vi "SerialArduino.vi"() -> ()   [LabVIEW 2019]
uses:
  96367c49-4912-4b9a-9665-363ed8841c2b.vi
  <vilib>/Instr/_visa.llb/VISA Configure Serial Port (Instr).vi
panel:
  out "return count":u32
  out "read buffer 2":string
  in  "Combo Box":string(combo)
  in  "stop":bool
  in  "Do Command":bool
  out "Result":dbl
  in  "Inputs":dbl[](array[numeric])
  out "error out":errorcluster
  out "read buffer":string
  in  "VISA resource name":refnum<visa-resource-name>
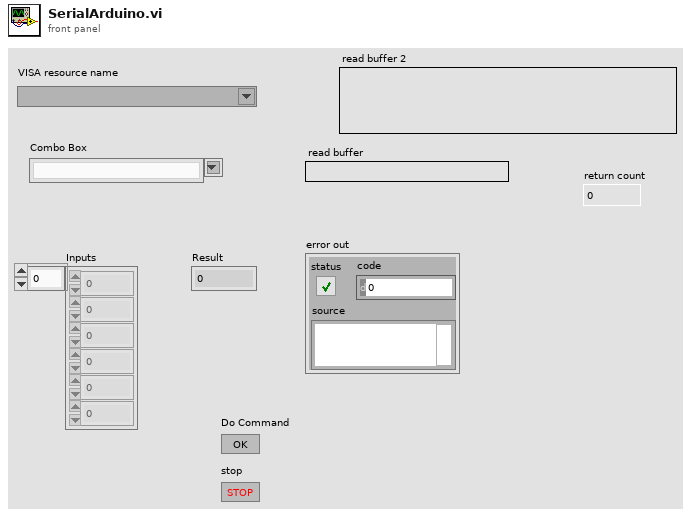
[diagram p1: front panel]
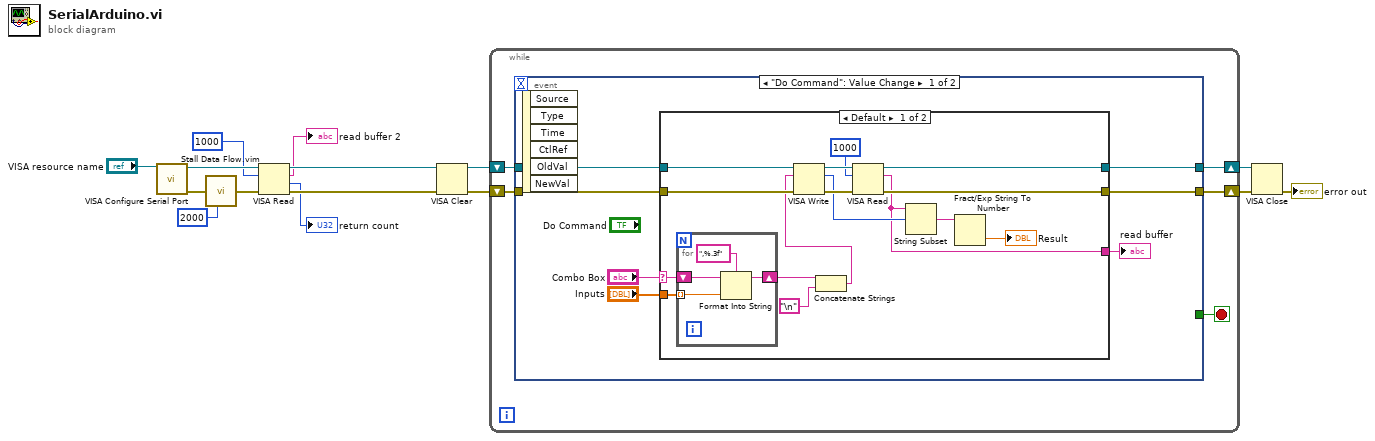
[diagram p0: block diagram]
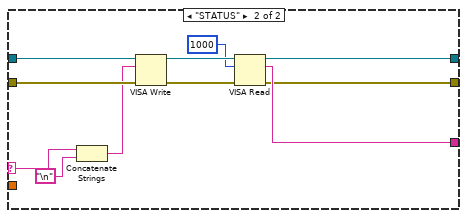
[diagram p2: hidden frame]
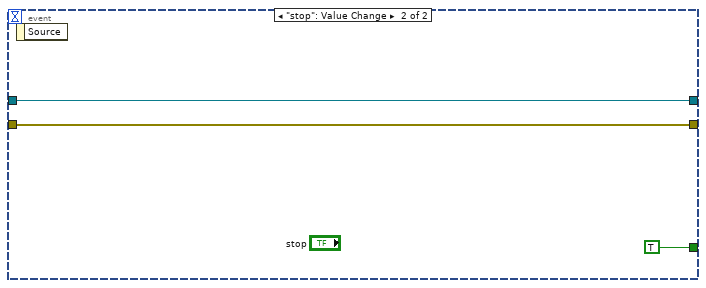
[diagram p3: hidden frame]
diagram:
  n1 = call-poly "VISA Configure Serial Port"("VISA resource name"="VISA resource name") -> ("VISA resource name out"=w5:refnum<visa-resource-name>, "error out"=w15:errorcluster)  [unwired: 13 in]
  n2 = call "Stall Data Flow.vim"("value in"=w15, "milliseconds to wait"=u32 2000) -> ("value out"=w8:errorcluster)  [unwired: 1 out]
  n3 = VISA Read(VISA resource name=w5, byte count=u32 1000, error in (no error)=w8) -> (VISA resource name out=w4:refnum<visa-resource-name>, read buffer=→"read buffer 2":string, return count=→"return count":u32, error out=w6:errorcluster)
  n4 = VISA Clear(VISA resource name=w4, error in (no error)=w6) -> (VISA resource name out=w14:refnum<visa-resource-name>, error out=w13:errorcluster)
  n5 = while {
    shift-right: [w18] -> w12
    shift-left: w14 -> [w20]
    shift-right: [w17] -> w11
    shift-left: w13 -> [w19]
    stop <- w16 stop-if-true
    n6 = event shown="[0] \"Do Command\": Value Change" {
      selector: _ -> [_ _]
      dyn-events: _ -> [_ _]
      timeout: _ -> [_ _]
      tunnel: w20 -> [w27 w60]
      tunnel: w19 -> [w26 w59]
      tunnel: [w25 w60] -> w18
      tunnel: [w24 w59] -> w17
      tunnel: [_ TRUE] -> w16
      event "Do Command": Value Change {
        n7 = event-data() -> ()  [unwired: 1 in, 6 out]
        n8 = case shown="Default" "Combo Box" {
          selector: "Combo Box" -> [w30 w50]
          tunnel: w27 -> [w43 w55]
          tunnel: w26 -> [w42 w54]
          tunnel: [w38 w51] -> w25
          tunnel: [w37 w52] -> w24
          tunnel: [w29 w53] -> w22
          tunnel: "Inputs" -> [w28 _]
          frame Default {
            n9 = for {
              shift-right: [w45] -> w36
              shift-left: w30 -> [w46]
              tunnel: w28 -> [w44] mode=indexing
              n10 = Format Into String(format string=",%.3f", initial string=w46, w44) -> (resulting string=w45:string)  [unwired: 1 in, 1 out]
            }
            n11 = Concatenate Strings(w36, "\n") -> (w34:string)
            n12 = VISA Write(VISA resource name=w43, write buffer=w34, error in (no error)=w42) -> (VISA resource name out=w41:refnum<visa-resource-name>, return count=w33:u32, error out=w40:errorcluster)
            n13 = VISA Read(VISA resource name=w41, byte count=u32 1000, error in (no error)=w40) -> (VISA resource name out=w38:refnum<visa-resource-name>, read buffer=w29:string, error out=w37:errorcluster)  [unwired: 1 out]
            n14 = String Subset(string=w29, offset (0)=w33) -> (substring=w32:string)  [unwired: 1 in]
            n15 = Fract/Exp String To Number(string=w32) -> (number=→"Result":dbl)  [unwired: 3 in, 1 out]
          }
          frame "STATUS" {
            n16 = Concatenate Strings(w50, "\n") -> (w49:string)
            n17 = VISA Write(VISA resource name=w55, write buffer=w49, error in (no error)=w54) -> (VISA resource name out=w58:refnum<visa-resource-name>, error out=w57:errorcluster)  [unwired: 1 out]
            n18 = VISA Read(VISA resource name=w58, byte count=u32 1000, error in (no error)=w57) -> (VISA resource name out=w51:refnum<visa-resource-name>, read buffer=w53:string, error out=w52:errorcluster)  [unwired: 1 out]
          }
        }
        "read buffer" <- w22
      }
      event "stop": Value Change {
        n19 = event-data() -> ()  [unwired: 1 in, 1 out]
      }
    }
  }
  n20 = VISA Close(VISA resource name=w12, error in (no error)=w11) -> (error out=→"error out":errorcluster)
